vi "instance count allowed.vi"(8 "error in":errorcluster, 11 "shared memory module configuration":refnum<class "Shared Memory Configuration.lvclass">) -> (0 "error out":errorcluster, 2 "instances allowed":i32, 3 "shared memory module configuration out":refnum<class "Shared Memory Configuration.lvclass">)   [LabVIEW 2013, in "Shared Memory Configuration.lvclass"]
uses:
  Shared Memory Configuration.lvclass
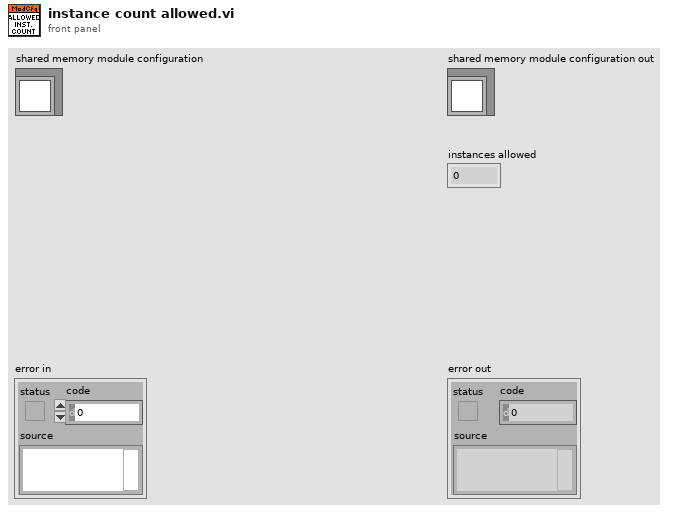
[diagram p1: front panel]
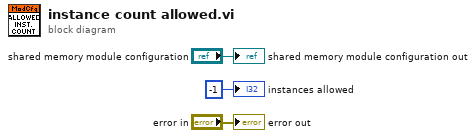
[diagram p0: block diagram]
diagram:
  "error out" <- "error in"
  "shared memory module configuration out" <- "shared memory module configuration"
  "instances allowed" <- -1 ("instances allowed")
